vi "Send Number.vi"(8 "error in":errorcluster, 9 "Number Numeric":dbl, 10 "Number String":string) -> (0 "error out":errorcluster)   [LabVIEW 2025, in "Number Pad.lvlib"]
doc: "Broadcast the number as a string and DBL to any listening module.\n\n_____\nCreated using DQMH Framework: Event Scripter 7.1.0.1503."
uses:
  Number Pad.lvlib
  Send Number Argument--cluster.ctl
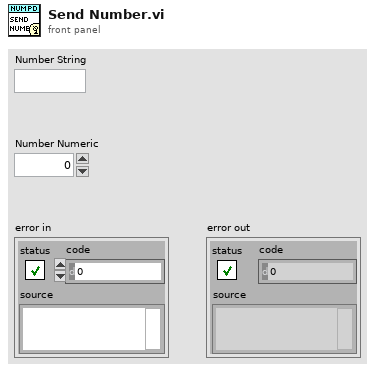
[diagram p1: front panel]
types:
  T1 = typedef "Number Pad.lvlib/Send Number Argument--cluster.ctl" = cluster{"Number String":string, "Number Numeric":dbl}
  T2 = typedef "Number Pad.lvlib/Broadcast Events--cluster.ctl" = cluster{"Module Did Init":refnum<user-event>, "Status Updated":refnum<user-event>, "Error Reported":refnum<user-event>, "Module Did Stop":refnum<user-event>, "Update Module Execution Status":refnum<user-event>, "Send Number":refnum<user-event>}
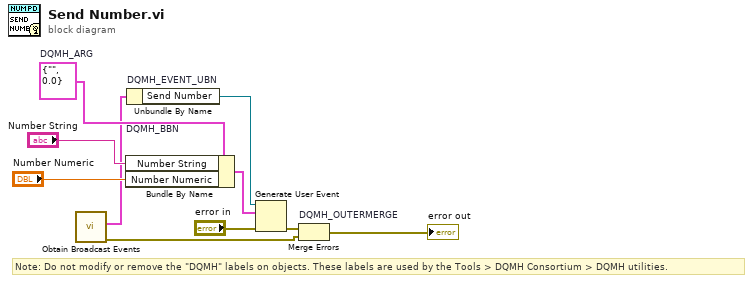
[diagram p0: block diagram]
diagram:
  w5 = T1 {"Number String"="", "Number Numeric"=0.0}  # DQMH_ARG
  # "Note: Do not modify or remove the \"DQMH\" labels on objects. These labels are used by the Tools > DQMH Consortium > DQMH utilities."
  n1 = call "Obtain Broadcast Events.vi"() -> ("error out"=w2:errorcluster, "Number Pad Broadcast Events"=w1:T2)  [unwired: 10 in]
  n2 = Bundle By Name "DQMH_BBN"(cluster=w5, "Number String"="Number String", "Number Numeric"="Number Numeric") -> (w8:T1)
  n3 = Unbundle By Name "DQMH_EVENT_UBN"(w1) -> ("Send Number"=w7:refnum<user-event>)
  n4 = Generate User Event(user event=w7, event data cluster=w8, error in="error in") -> (error out=w6:errorcluster)  [unwired: 1 in, 1 out]
  n5 = Merge Errors "DQMH_OUTERMERGE"(w6, w2) -> (→"error out":errorcluster)
